vi "Calculate Velocity Setpoints.vi"(6 "IMU Input":dbl, 8 "Iterations":i32, 9 "Angular Data (Relative)":dbl[](array[numeric]), 10 "Velocity Data":dbl[](array[numeric]), 11 "Enum":enum16{"JV", "Mule", "Linda/Sophie"}(ring)) -> (1 "Finished?":bool, 2 "Right Setpoint":dbl, 3 "Left Setpoint":dbl)   [LabVIEW 2019]
uses:
  <vilib>/addons/control/pid/pid.llb/PID (DBL).vi
  <vilib>/addons/control/pid/NI_PID_pid.lvlib
panel:
  out "Angles PID":cluster{"IPCed":dbl, "output 2":dbl}
  in  "PID gains":T1={"proportional gain (Kc)"=0.02, "integral time (Ti, min)"=0.001, "derivative time (Td, min)"=0.0} {"derivative time (Td, min)" format="%.3f"; "integral time (Ti, min)" format="%.3f"; "proportional gain (Kc)" format="%.3f"}
  in  "Angle To Get":dbl(slide) scale=0.0..360.0
  in  "Align?":bool
  out "Timing Feedback":u32(graph)
  out "Wait Time (ms)":dbl
  out "Angles PID L/S":cluster{"Numeric":dbl, "IMU Input":dbl}(graph)
  in  "f":dbl=0.17 format="%#_13g"
  in  "PID gains L/S 2":T1={"proportional gain (Kc)"=0.08, "integral time (Ti, min)"=0.0, "derivative time (Td, min)"=0.001} {"derivative time (Td, min)" format="%.3e"; "integral time (Ti, min)" format="%.3e"; "proportional gain (Kc)" format="%#.6e"}
  out "Angles PID M":cluster{"Numeric":dbl, "IMU Input":dbl}(graph)
  in  "Time":u32
  in  "Front is Back":bool
  in  "Reversed":bool
  in  "Negated":bool
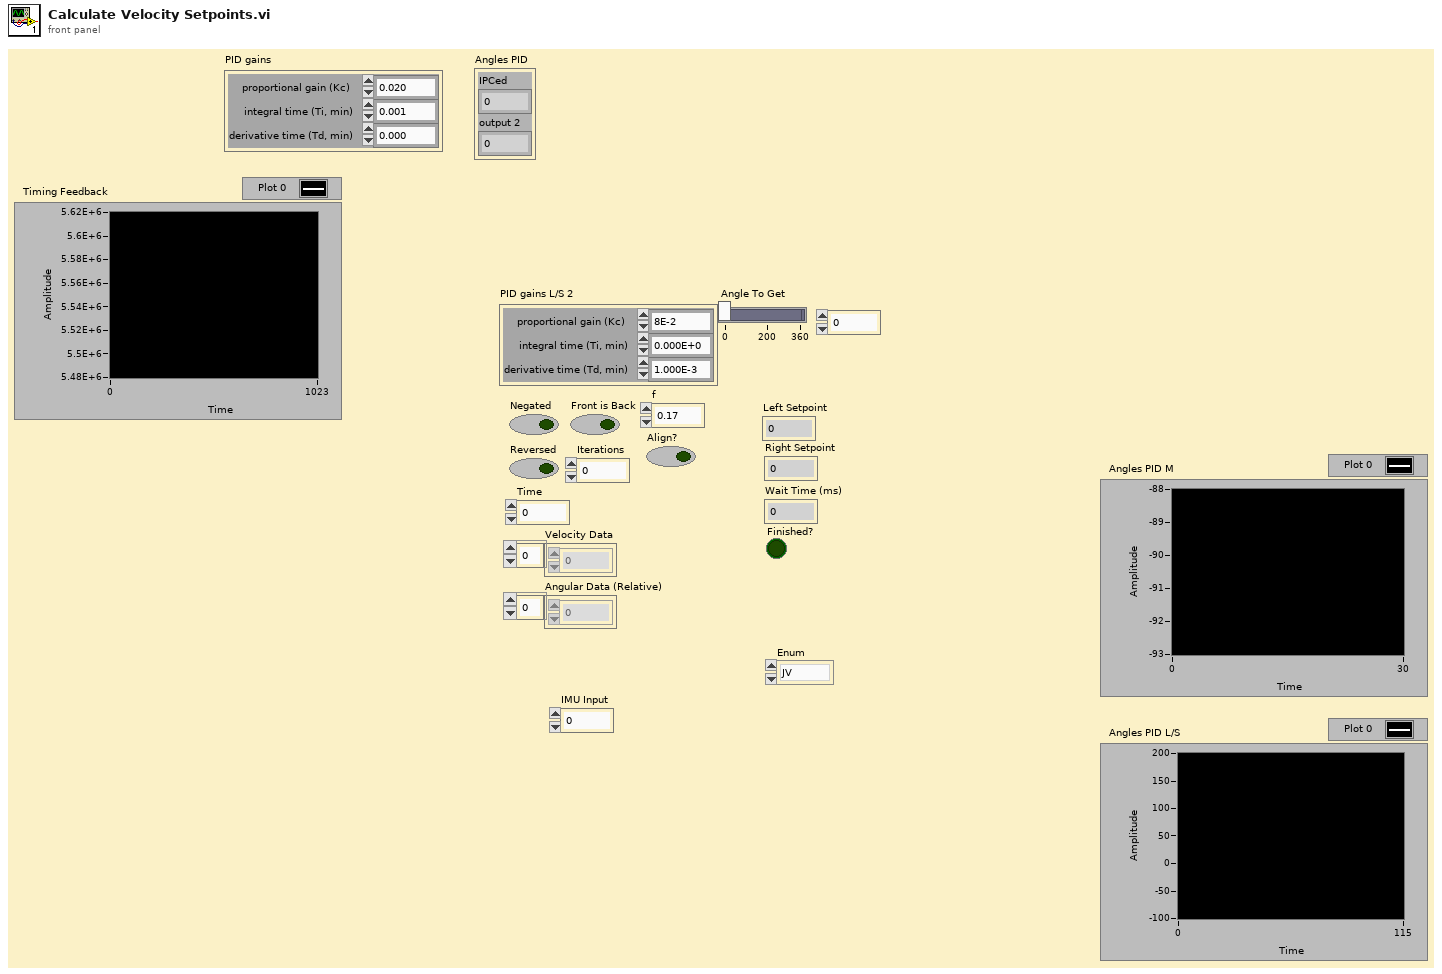
[diagram p1: front panel]
types:
  T1 = cluster{"proportional gain (Kc)":dbl, "integral time (Ti, min)":dbl, "derivative time (Td, min)":dbl}
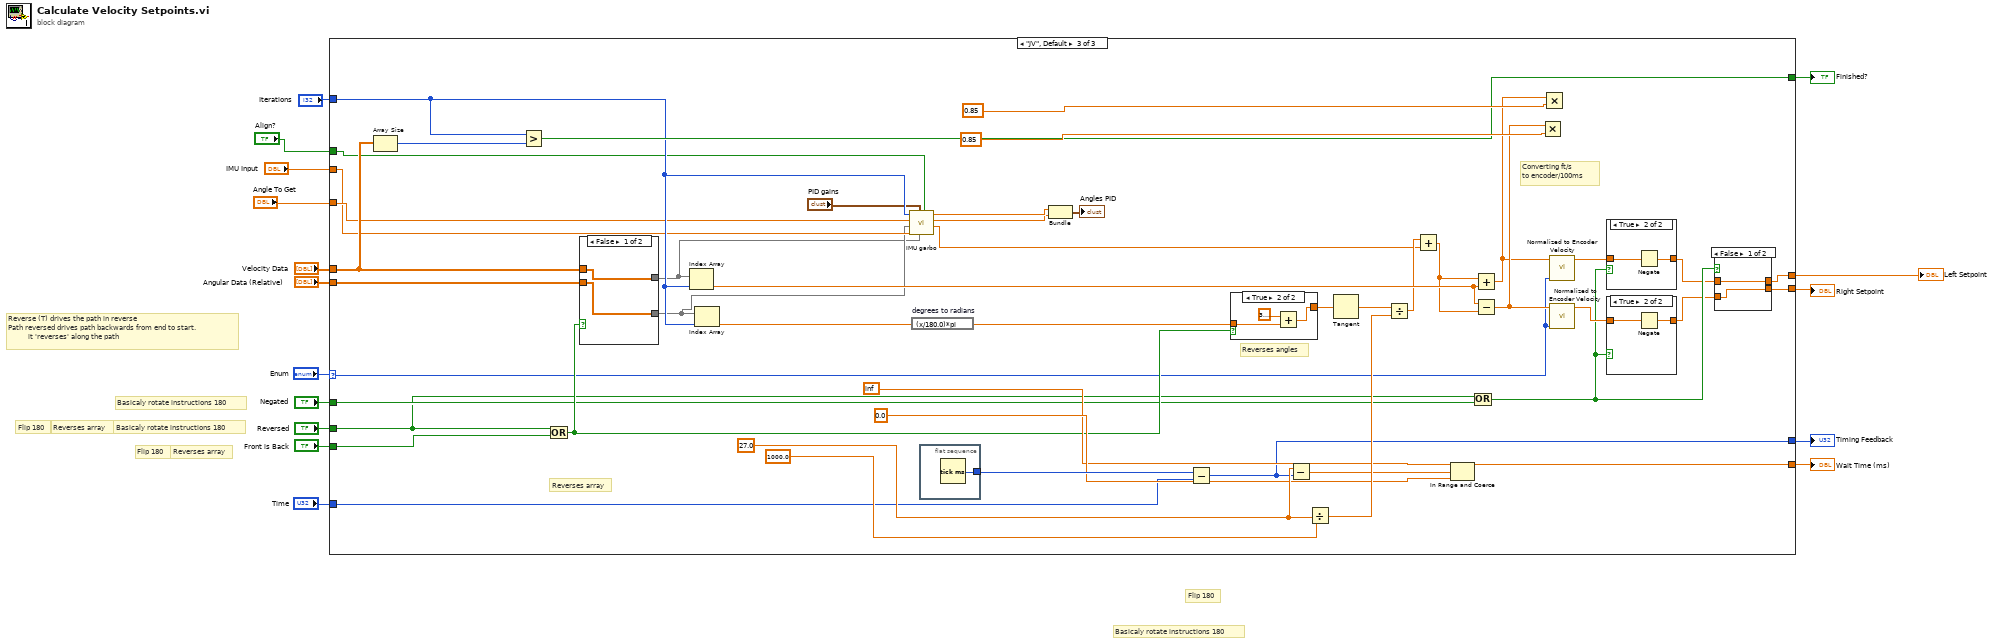
[diagram p0: block diagram]
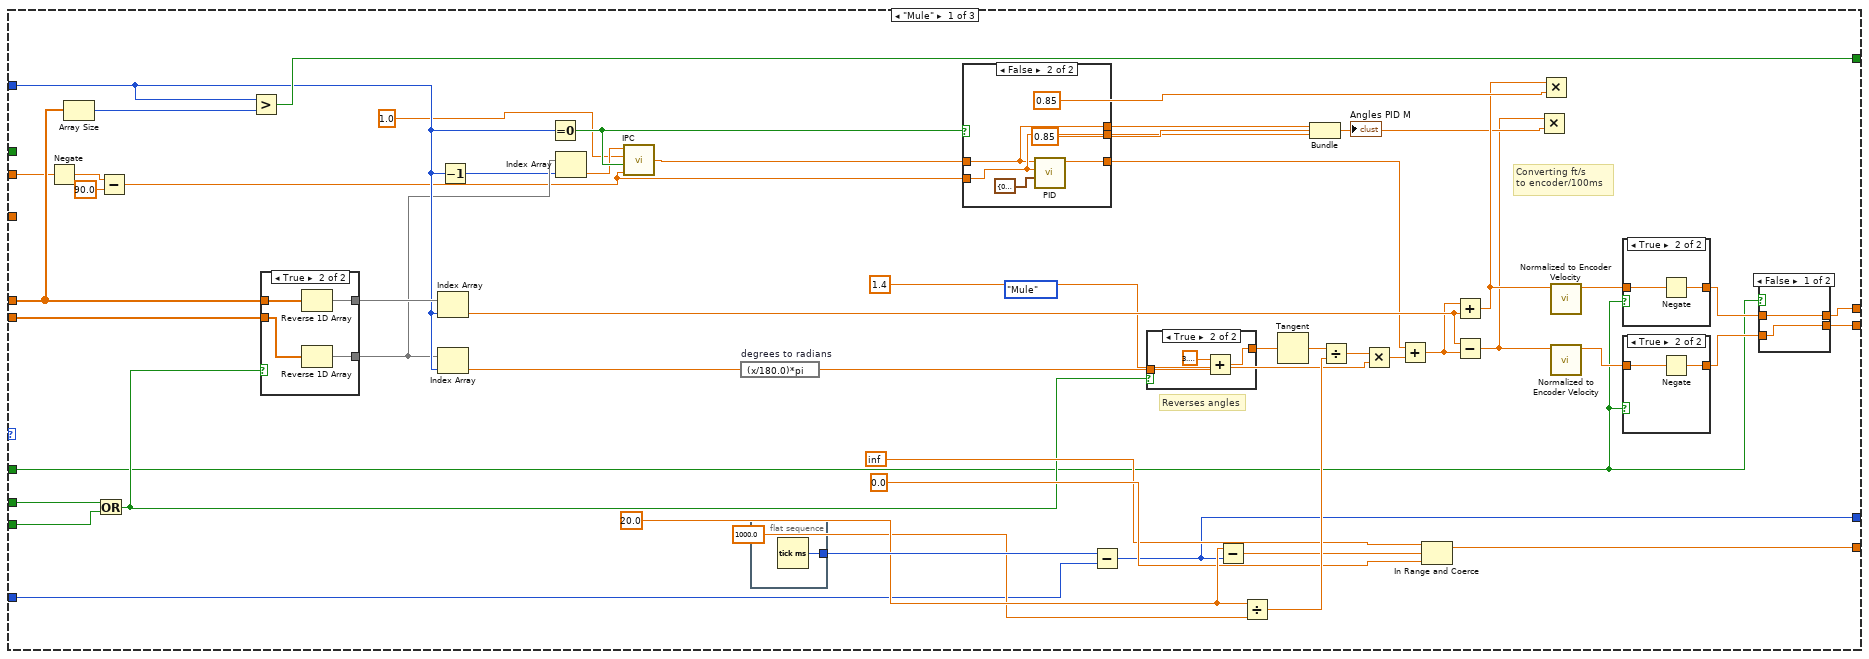
[diagram p2: hidden frame]
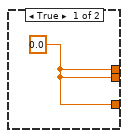
[diagram p3: hidden frame]
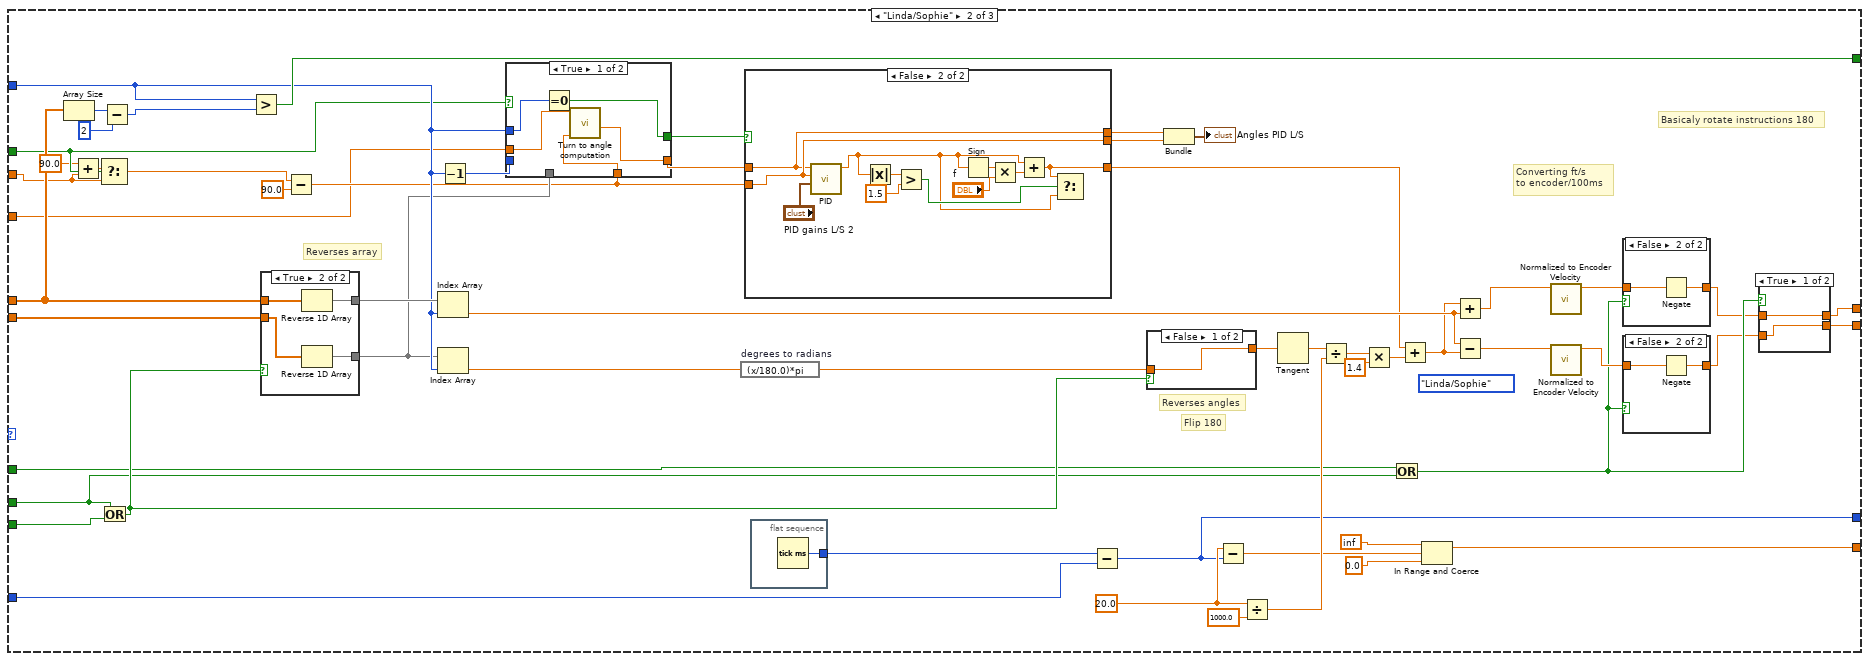
[diagram p9: hidden frame]
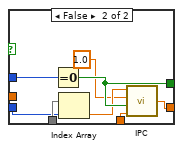
[diagram p10: hidden frame]
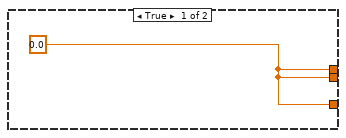
[diagram p11: hidden frame]
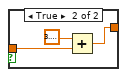
[diagram p14: hidden frame]
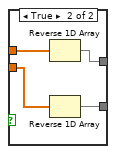
[diagram p18: hidden frame]
diagram:
  # "Reverse (T) drives the path in reverse\nPath reversed drives path backwards from end to start. \n          it 'reverses' along the path"
  # "Basicaly rotate instructions 180"
  # "Basicaly rotate instructions 180"
  # "Flip 180"
  # "Flip 180"
  # "Reverses array"
  # "Reverses array"
  # "Flip 180"
  # "Basicaly rotate instructions 180"
  n1 = case shown="\"JV\", Default" "Enum" {
    selector: "Enum" -> [_ _ w212]
    tunnel: "Negated" -> [w17 w135 w227]
    tunnel: "Reversed" -> [w53 w134 w226]
    tunnel: "Front is Back" -> [w52 w133 w225]
    tunnel: "Iterations" -> [w26 w112 w208]
    tunnel: "Time" -> [w51 w132 w224]
    tunnel: "Angular Data (Relative)" -> [w50 w131 w223]
    tunnel: "Velocity Data" -> [w49 w130 w222]
    tunnel: [w44 w127 w218] -> w8
    tunnel: [w43 w126 w217] -> w3
    tunnel: [w42 w125 w216] -> w7
    tunnel: [w41 w124 w215] -> w6
    tunnel: [w40 w123 w214] -> w5
    tunnel: "IMU Input" -> [w29 w98 w206]
    tunnel: "Align?" -> [_ w101 w203]
    tunnel: "Angle To Get" -> [_ w102 w207]
    frame "Mule" {
      (unwired) enum16{"Vantage", "Mule"}."Mule" ("Enum")
      w67 = 20.0 ("x")
      # "Converting ft/s\nto encoder/100ms"
      # "Reverses angles"
      n2 = Negate(x=w29) -> (-x=w28:dbl)
      n3 = Array Size(array=w49) -> (size(s)=w57:i32)
      n4 = Or(x=w53, y=w52) -> (x .or. y?=w56:bool)
      n5 = Subtract(x=w28, y=90.0) -> (x-y=w20:dbl)
      n6 = Greater?(x=w26, y=w57) -> (0:w40:bool)
      n7 = case shown="True" w56 {
        tunnel: [w79 w84] -> w25
        tunnel: [w80 w83] -> w58
        tunnel: w50 -> [w79 w81]
        tunnel: w49 -> [w80 w82]
        frame False {
        }
        frame True {
          n8 = Reverse 1D Array(array=w82) -> (reversed array=w83:dbl[])
          n9 = Reverse 1D Array(array=w81) -> (reversed array=w84:dbl[])
        }
      }
      n10 = Index Array(array=w58, index=w26) -> (element=w39:dbl)
      n11 = Index Array(array=w25, index=w26) -> (element=w37:dbl)
      n12 = Decrement(x=w26) -> (x-1=w24:i32)
      n13 = Equal To 0?(x=w26) -> (x = 0?=w23:bool)
      n14 = Index Array(array=w25, index=w24) -> (element=w22:dbl)
      n15 = call "IPC.vi"("Initilization"=w20, "Reset"=w23, "Multiplier"=1.0, "Value"=w22) -> ("IPCed"=w21:dbl)  [unwired: 2 in]
      n16 = expression code="(x/180.0)*pi" "degrees to radians"(w37) -> (w36:dbl)
      n17 = flat-sequence {
        tunnel: [w95] -> w69
        frame #0 {
          n18 = Tick Count (ms)() -> (millisecond timer value=w95:u32)
        }
      }
      n19 = case shown="False" w23 {
        tunnel: w20 -> [_ w72]
        tunnel: [w70 w73] -> w18
        tunnel: [w70 w71] -> w31
        tunnel: [w70 w72] -> w30
        tunnel: w21 -> [_ w71]
        frame True {
          w70 = 0.0 ("output")
        }
        frame False {
          n20 = call-poly <vilib>:"PID.vi"("PID gains"=T1 {"proportional gain (Kc)"=0.2, "integral time (Ti, min)"=0.4, "derivative time (Td, min)"=0.0006} ("PID gains M"), "process variable"=w72, "setpoint"=w71) -> ("output"=w73:dbl)  [unwired: 7 in, 1 out]
        }
      }
      n21 = Subtract(x=w69, y=w51) -> (x-y=w41:u32)
      n22 = case shown="True" w56 {
        tunnel: w36 -> [w85 w88]
        tunnel: [w85 w87] -> w59
        frame False {
        }
        frame True {
          n23 = Add(x=3.141592653589793, y=w88) -> (x+y=w87:dbl)
        }
      }
      n24 = Subtract(x=w67, y=w41) -> (x-y=w63:dbl)
      n25 = Divide(x=w67, y=1000.0) -> (x/y=w65:dbl)
      n26 = Tangent(1:w59) -> (0:w68:dbl)
      n27 = Bundle("IPCed"=w31, "output"=w30) -> (→"Angles PID M":cluster{"IPCed":dbl, "output":dbl})  [unwired: 1 in]
      n28 = Divide(x=w68, y=w65) -> (x/y=w38:dbl)
      n29 = Multiply(x=w38, y=1.4) -> (x*y=w34:dbl)
      n30 = Add(x=w18, y=w34) -> (x+y=w33:dbl)
      n31 = In Range and Coerce(upper limit=inf, x=w63, lower limit=0.0) -> (coerced(x)=w42:dbl)  [unwired: 1 out]
      n32 = Add(x=w33, y=w39) -> (x+y=w47:dbl)
      n33 = Subtract(x=w39, y=w33) -> (x-y=w45:dbl)
      n34 = Multiply(x=w45, y=0.85) -> ()  [unwired: 1 out]
      n35 = Multiply(x=w47, y=0.85) -> ()  [unwired: 1 out]
      n36 = call "Normalized to Encoder Velocity.vi"("ft/s"=w47) -> ("Output"=w61:dbl)  [unwired: 10 in]
      n37 = call "Normalized to Encoder Velocity.vi"("ft/s"=w45) -> ("Output"=w60:dbl)  [unwired: 10 in]
      n38 = case shown="True" w17 {
        tunnel: w61 -> [w92 w94]
        tunnel: [w92 w93] -> w55
        frame False {
        }
        frame True {
          n39 = Negate(x=w94) -> (-x=w93:dbl)
        }
      }
      n40 = case shown="True" w17 {
        tunnel: [w89 w91] -> w54
        tunnel: w60 -> [w89 w90]
        frame False {
        }
        frame True {
          n41 = Negate(x=w90) -> (-x=w91:dbl)
        }
      }
      n42 = case shown="False" w17 {
        tunnel: w54 -> [w76 w77]
        tunnel: w55 -> [w75 w78]
        tunnel: [w76 w78] -> w44
        tunnel: [w75 w77] -> w43
        frame False {
        }
        frame True {
        }
      }
    }
    frame "Linda/Sophie" {
      (unwired) enum16{"Vantage", "Mule", "Linda/Sophie"}."Linda/Sophie" ("Enum")
      w149 = 20.0 ("x")
      # "Basicaly rotate instructions 180"
      # "Flip 180"
      # "Reverses array"
      # "Converting ft/s\nto encoder/100ms"
      # "Reverses angles"
      n43 = Array Size(array=w130) -> (size(s)=w105:i32)
      n44 = Add(x=90.0, y=w98) -> (x+y=w99:dbl)
      n45 = Select(t=w99, s=w101, f=w98) -> (s? t:f=w96:dbl)
      n46 = Or(x=w134, y=w133) -> (x .or. y?=w139:bool)
      n47 = Subtract(x=w105, y=2) -> (x-y=w104:i32)
      n48 = Greater?(x=w112, y=w104) -> (0:w123:bool)
      n49 = case shown="True" w139 {
        tunnel: [w181 w186] -> w111
        tunnel: [w182 w185] -> w140
        tunnel: w131 -> [w181 w183]
        tunnel: w130 -> [w182 w184]
        frame False {
        }
        frame True {
          n50 = Reverse 1D Array(array=w184) -> (reversed array=w185:dbl[])
          n51 = Reverse 1D Array(array=w183) -> (reversed array=w186:dbl[])
        }
      }
      n52 = Subtract(x=w96, y=90.0) -> (x-y=w107:dbl)
      n53 = Index Array(array=w140, index=w112) -> (element=w122:dbl)
      n54 = Index Array(array=w111, index=w112) -> (element=w120:dbl)
      n55 = Decrement(x=w112) -> (x-1=w110:i32)
      n56 = case shown="True" w101 {
        tunnel: w112 -> [w153 w164]
        tunnel: w111 -> [_ w163]
        tunnel: w110 -> [_ w162]
        tunnel: [w152 w161] -> w109
        tunnel: [w154 w159] -> w108
        tunnel: w107 -> [w156 w158]
        tunnel: w102 -> [w155 _]
        frame True {
          n57 = Equal To 0?(x=w153) -> (x = 0?=w152:bool)
          n58 = call "Turn to angle computation.vi"("Current Angle"=w156, "Angle To Get"=w155) -> ("Current Angle 2"=w154:dbl)  [unwired: 9 in]
        }
        frame False {
          n59 = Equal To 0?(x=w164) -> (x = 0?=w161:bool)
          n60 = Index Array(array=w163, index=w162) -> (element=w160:dbl)
          n61 = call "IPC.vi"("Initilization"=w158, "Reset"=w161, "Multiplier"=1.0, "Value"=w160) -> ("IPCed"=w159:dbl)  [unwired: 2 in]
        }
      }
      n62 = expression code="(x/180.0)*pi" "degrees to radians"(w120) -> (w119:dbl)
      n63 = case shown="False" w109 {
        tunnel: w107 -> [_ w176]
        tunnel: [w165 w169] -> w106
        tunnel: [w165 w175] -> w114
        tunnel: [w165 w176] -> w113
        tunnel: w108 -> [_ w175]
        frame True {
          w165 = 0.0 ("output")
        }
        frame False {
          n64 = call-poly <vilib>:"PID.vi"("PID gains"="PID gains L/S 2", "process variable"=w176, "setpoint"=w175) -> ("output"=w167:dbl)  [unwired: 7 in, 1 out]
          n65 = Absolute Value(x=w167) -> (abs(x)=w171:dbl)
          n66 = Greater?(x=w171, y=1.5) -> (0:w168:bool)
          n67 = Sign(1:w167) -> (0:w174:dbl)
          n68 = Multiply(x=w174, y="f") -> (x*y=w173:dbl)
          n69 = Add(x=w167, y=w173) -> (x+y=w169:dbl)
          n70 = Select(t=w169, s=w168, f=w167) -> ()  [unwired: 1 out]
        }
      }
      n71 = flat-sequence {
        tunnel: [w197] -> w151
        frame #0 {
          n72 = Tick Count (ms)() -> (millisecond timer value=w197:u32)
        }
      }
      n73 = Subtract(x=w151, y=w132) -> (x-y=w124:u32)
      n74 = case shown="False" w139 {
        tunnel: w119 -> [w187 w190]
        tunnel: [w187 w189] -> w141
        frame False {
        }
        frame True {
          n75 = Add(x=3.141592653589793, y=w190) -> (x+y=w189:dbl)
        }
      }
      n76 = Bundle("IPCed"=w114, "output"=w113) -> (→"Angles PID L/S":cluster{"IPCed":dbl, "output":dbl})  [unwired: 1 in]
      n77 = Subtract(x=w149, y=w124) -> (x-y=w145:dbl)
      n78 = Divide(x=w149, y=1000.0) -> (x/y=w147:dbl)
      n79 = Tangent(1:w141) -> (0:w150:dbl)
      n80 = Divide(x=w150, y=w147) -> (x/y=w121:dbl)
      n81 = Multiply(x=w121, y=1.4) -> (x*y=w117:dbl)
      n82 = Or(x=w135, y=w134) -> (x .or. y?=w138:bool)
      n83 = Add(x=w106, y=w117) -> (x+y=w116:dbl)
      n84 = In Range and Coerce(upper limit=inf, x=w145, lower limit=0.0) -> (coerced(x)=w125:dbl)  [unwired: 1 out]
      n85 = Add(x=w116, y=w122) -> (x+y=w129:dbl)
      n86 = Subtract(x=w122, y=w116) -> (x-y=w128:dbl)
      n87 = call "Normalized to Encoder Velocity.vi"("ft/s"=w129) -> ("Output"=w143:dbl)  [unwired: 10 in]
      n88 = call "Normalized to Encoder Velocity.vi"("ft/s"=w128) -> ("Output"=w142:dbl)  [unwired: 10 in]
      n89 = case shown="False" w138 {
        tunnel: w143 -> [w194 w196]
        tunnel: [w194 w195] -> w137
        frame True {
        }
        frame False {
          n90 = Negate(x=w196) -> (-x=w195:dbl)
        }
      }
      n91 = case shown="False" w138 {
        tunnel: [w191 w193] -> w136
        tunnel: w142 -> [w191 w192]
        frame True {
        }
        frame False {
          n92 = Negate(x=w192) -> (-x=w193:dbl)
        }
      }
      n93 = case shown="True" w138 {
        tunnel: w136 -> [w178 w179]
        tunnel: w137 -> [w177 w180]
        tunnel: [w178 w180] -> w127
        tunnel: [w177 w179] -> w126
        frame True {
        }
        frame False {
        }
      }
    }
    frame "JV", Default {
      w242 = 27.0 ("x")
      # "Reverses array"
      # "Converting ft/s\nto encoder/100ms"
      # "Reverses angles"
      n94 = Array Size(array=w222) -> (size(s)=w232:i32)
      n95 = Greater?(x=w208, y=w232) -> (0:w214:bool)
      n96 = Or(x=w226, y=w225) -> (x .or. y?=w231:bool)
      n97 = case shown="False" w231 {
        tunnel: [w250 w255] -> w205
        tunnel: [w251 w254] -> w204
        tunnel: w223 -> [w250 w252]
        tunnel: w222 -> [w251 w253]
        frame False {
        }
        frame True {
          n98 = Reverse 1D Array(array=w253) -> (reversed array=w254:dbl[])
          n99 = Reverse 1D Array(array=w252) -> (reversed array=w255:dbl[])
        }
      }
      n100 = Index Array(array=w204, index=w208) -> (element=w244:dbl)
      n101 = Index Array(array=w205, index=w208) -> (element=w211:dbl)
      n102 = call "IMU garbo.vi"("Align?"=w203, "Velocity Data"=w204, "PID gains"="PID gains", "Numeric"=w206, "Angular Data (Relative)"=w205, "Angle to Get"=w207, "Iterations"=w208) -> ("output"=w198:dbl, "output 2"=w200:dbl, "IPCed"=w201:dbl)  [unwired: 1 in, 1 out]
      n103 = expression code="(x/180.0)*pi" "degrees to radians"(w211) -> (w234:dbl)
      n104 = flat-sequence {
        tunnel: [w266] -> w245
        frame #0 {
          n105 = Tick Count (ms)() -> (millisecond timer value=w266:u32)
        }
      }
      n106 = Bundle("IPCed"=w201, "output 2"=w200) -> (→"Angles PID":cluster{"IPCed":dbl, "output 2":dbl})  [unwired: 1 in]
      n107 = Subtract(x=w245, y=w224) -> (x-y=w215:u32)
      n108 = case shown="True" w231 {
        tunnel: w234 -> [w256 w259]
        tunnel: [w256 w258] -> w233
        frame False {
        }
        frame True {
          n109 = Add(x=3.141592653589793, y=w259) -> (x+y=w258:dbl)
        }
      }
      n110 = Subtract(x=w242, y=w215) -> (x-y=w238:dbl)
      n111 = Divide(x=w242, y=1000.0) -> (x/y=w240:dbl)
      n112 = Tangent(1:w233) -> (0:w243:dbl)
      n113 = Divide(x=w243, y=w240) -> (x/y=w210:dbl)
      n114 = Add(x=w210, y=w198) -> (x+y=w209:dbl)
      n115 = In Range and Coerce(upper limit=inf, x=w238, lower limit=0.0) -> (coerced(x)=w216:dbl)  [unwired: 1 out]
      n116 = Or(x=w226, y=w227) -> (x .or. y?=w230:bool)
      n117 = Add(x=w209, y=w244) -> (x+y=w213:dbl)
      n118 = Subtract(x=w244, y=w209) -> (x-y=w219:dbl)
      n119 = Multiply(x=w219, y=0.85) -> ()  [unwired: 1 out]
      n120 = Multiply(x=w213, y=0.85) -> ()  [unwired: 1 out]
      n121 = call "Normalized to Encoder Velocity.vi"("Enum"=w212, "ft/s"=w213) -> ("Output"=w236:dbl)  [unwired: 9 in]
      n122 = call "Normalized to Encoder Velocity.vi"("Enum"=w212, "ft/s"=w219) -> ("Output"=w235:dbl)  [unwired: 9 in]
      n123 = case shown="True" w230 {
        tunnel: w236 -> [w263 w265]
        tunnel: [w263 w264] -> w229
        frame False {
        }
        frame True {
          n124 = Negate(x=w265) -> (-x=w264:dbl)
        }
      }
      n125 = case shown="True" w230 {
        tunnel: [w260 w262] -> w228
        tunnel: w235 -> [w260 w261]
        frame False {
        }
        frame True {
          n126 = Negate(x=w261) -> (-x=w262:dbl)
        }
      }
      n127 = case shown="False" w230 {
        tunnel: w228 -> [w247 w248]
        tunnel: w229 -> [w246 w249]
        tunnel: [w247 w249] -> w218
        tunnel: [w246 w248] -> w217
        frame False {
        }
        frame True {
        }
      }
    }
  }
  "Left Setpoint" <- w3
  "Right Setpoint" <- w8
  "Wait Time (ms)" <- w7
  "Timing Feedback" <- w6
  "Finished?" <- w5
